vi "RW Properties Engine.vi"(7 "File Action [Read]":enum16{"Read", "Write"}(ring), 8 "error in":errorcluster, 9 "Methods[]":T1(array[cluster]), 10 "Properties[]":T2(array[cluster]), 11 "Classes[]":T3(array[cluster])) -> (0 "error out":errorcluster, 1 "Methods Out":T1(array[cluster]), 2 "Properties Out":T2(array[cluster]), 3 "Classes Out":T3(array[cluster]), 4 "data missing?":bool, 6 "Data format changed":bool)   [LabVIEW 2023]
doc: "Gets data from shift register or from file. If format has changed, files may be out of date and VI will return empty arrays plus boolean indicating that data is missing, so it can be rebuilt."
panel:
  # "IN"
  # "OUT"
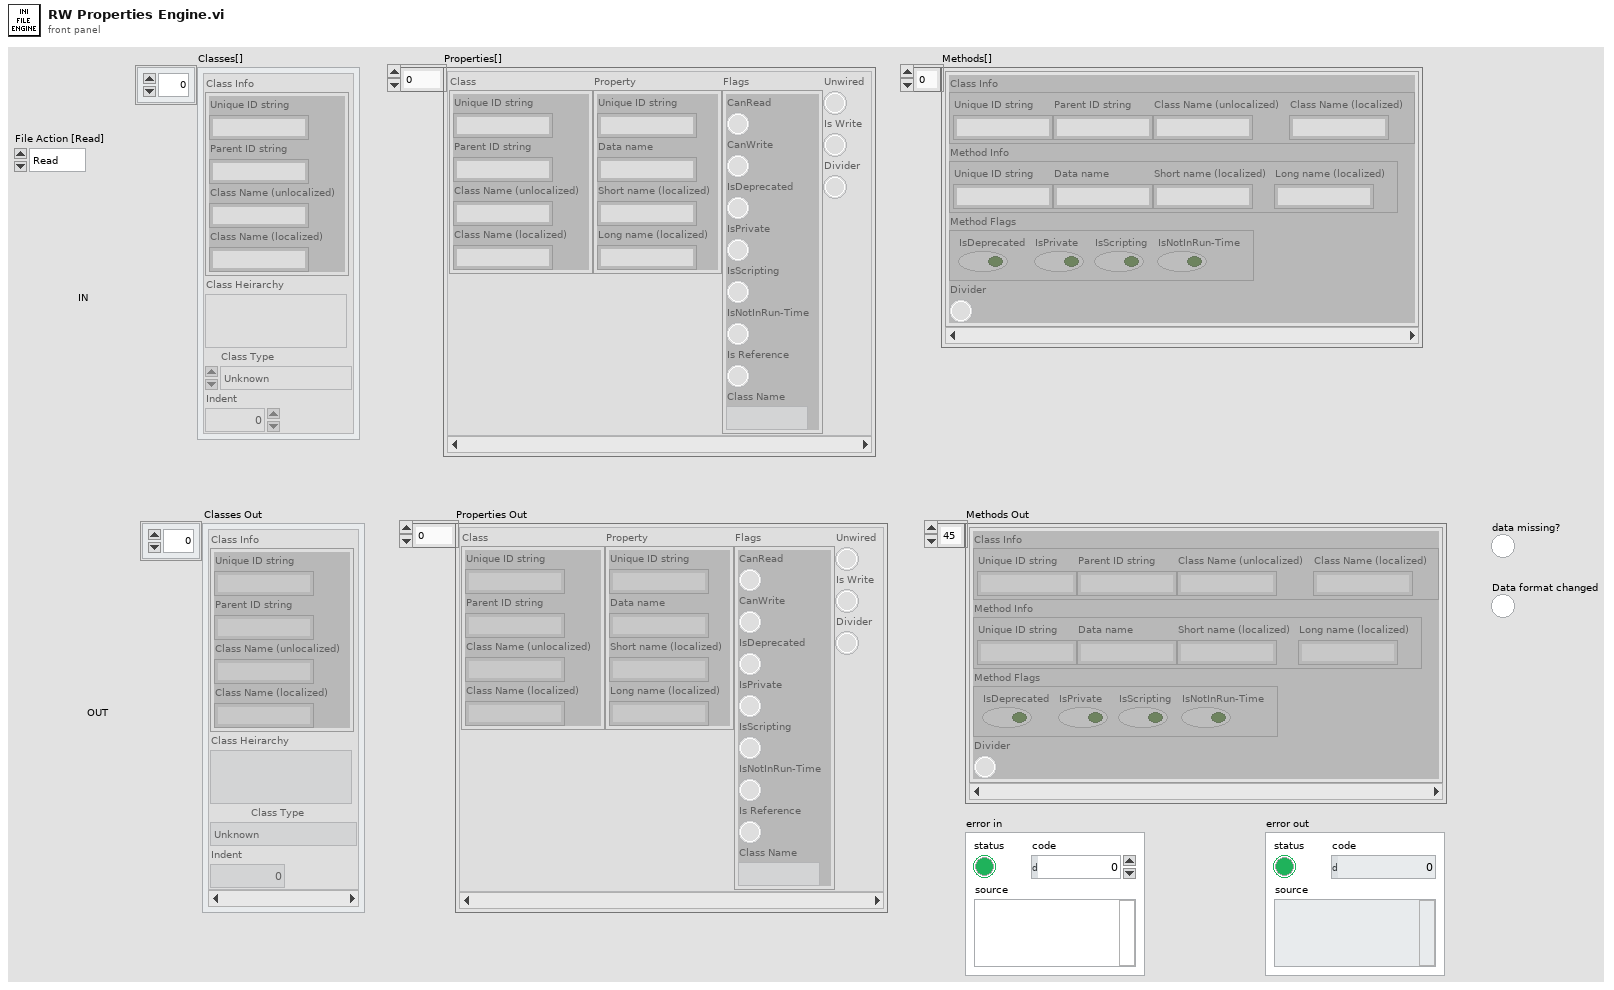
[diagram p1: front panel]
types:
  T1 = cluster{"Class Info":cluster{"Unique ID string":string, "Parent ID string":string, "Class Name (unlocalized)":string, "Class Name (localized)":string}, "Method Info":cluster{"Unique ID string":string, "Data name":string, "Short name (localized)":string, "Long name (localized)":string}, "Method Flags":cluster{"IsDeprecated":bool, "IsPrivate":bool, "IsScripting":bool, "IsNotInRun-Time":bool}, "Divider":bool}[]
  T2 = cluster{"Class":cluster{"Unique ID string":string, "Parent ID string":string, "Class Name (unlocalized)":string, "Class Name (localized)":string}, "Property":cluster{"Unique ID string":string, "Data name":string, "Short name (localized)":string, "Long name (localized)":string}, "Flags":cluster{"CanRead":bool, "CanWrite":bool, "IsDeprecated":bool, "IsPrivate":bool, "IsScripting":bool, "IsNotInRun-Time":bool, "Is Reference":bool, "Class Name":string}, "Divider":bool, "Is Write":bool, "Unwired":bool}[]
  T3 = cluster{"Class Info":cluster{"Unique ID string":string, "Parent ID string":string, "Class Name (unlocalized)":string, "Class Name (localized)":string}, "Class Heirarchy":string, "Class Type":enum16{"Unknown", "Base", "Scripting", "Private", "Deprecated", "None", "Divider"}, "Indent":u32}[]
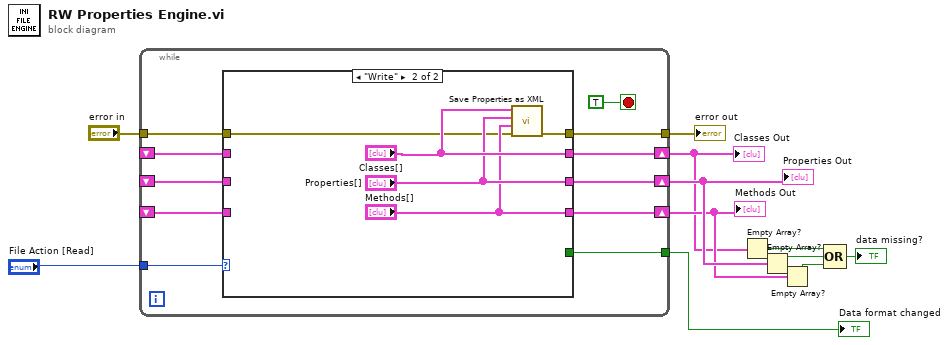
[diagram p0: block diagram]
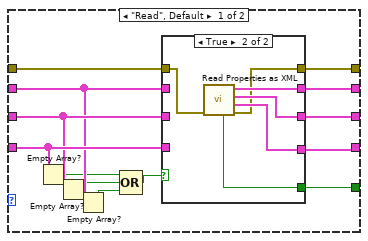
[diagram p2: hidden frame]
diagram:
  n1 = while {
    tunnel: "File Action [Read]" -> [w22]
    shift-right: [w20] -> w4
    shift-left: _ -> [w17]
    shift-right: [w19] -> w8
    shift-left: _ -> [w16]
    shift-right: [w18] -> w7
    shift-left: _ -> [w15]
    tunnel: [w14] -> w3
    tunnel: "error in" -> [w13]
    tunnel: [w12] -> w1
    stop <- TRUE stop-if-true
    n2 = case shown="\"Write\"" w22 {
      tunnel: [w35 "Classes[]"] -> w20
      tunnel: [w34 "Properties[]"] -> w19
      tunnel: [w33 "Methods[]"] -> w18
      tunnel: w17 -> [w30 _]
      tunnel: w16 -> [w31 _]
      tunnel: w15 -> [w32 _]
      tunnel: [w25 _] -> w14
      tunnel: w13 -> [w24 w47]
      tunnel: [w23 w46] -> w12
      frame "Read", Default {
        n3 = Empty Array?(array=w32) -> (empty?=w29:bool)
        n4 = Empty Array?(array=w31) -> (empty?=w28:bool)
        n5 = Empty Array?(array=w30) -> (empty?=w27:bool)
        n6 = Compound Arithmetic op=OR(w29, w28, w27) -> (w26:bool)
        n7 = case shown="True" w26 {
          tunnel: [w39 w45] -> w35
          tunnel: [w38 w44] -> w34
          tunnel: [w37 w43] -> w33
          tunnel: w30 -> [w39 _]
          tunnel: w31 -> [w38 _]
          tunnel: w32 -> [w37 _]
          tunnel: [_ w42] -> w25
          tunnel: w24 -> [w36 w41]
          tunnel: [w36 w40] -> w23
          frame False {
          }
          frame True {
            n8 = call "Read Properties as XML.vi"("error in"=w41) -> ("error out"=w40:errorcluster, "Methods[]"=w43:T1, "Properties[]"=w44:T2, "Classes"=w45:T3, "Data format changed"=w42:bool)  [unwired: 6 in]
          }
        }
      }
      frame "Write" {
        n9 = call "Save Properties as XML.vi"("error in"=w47, "Methods[]"="Methods[]", "Properties[]"="Properties[]", "Classes"="Classes[]") -> ("error out"=w46:errorcluster)  [unwired: 7 in]
      }
    }
  }
  "Properties Out" <- w8
  "Methods Out" <- w7
  "Classes Out" <- w4
  "Data format changed" <- w3
  "error out" <- w1
  n10 = Empty Array?(array=w4) -> (empty?=w9:bool)
  n11 = Empty Array?(array=w8) -> (empty?=w10:bool)
  n12 = Empty Array?(array=w7) -> (empty?=w11:bool)
  n13 = Compound Arithmetic op=OR(w9, w10, w11) -> (→"data missing?":bool)
